vi "Day 7.vi"() -> ()   [LabVIEW 2021]
uses:
  <vilib>/Utility/file.llb/Read Delimited Spreadsheet (I64).vi
panel:
  out "Min Position":i32
  out "Input":i64[](array[numeric])
  out "Solution Min Fuel":i32
  in  "Input File":enum32{"example input", "input"}(radio)
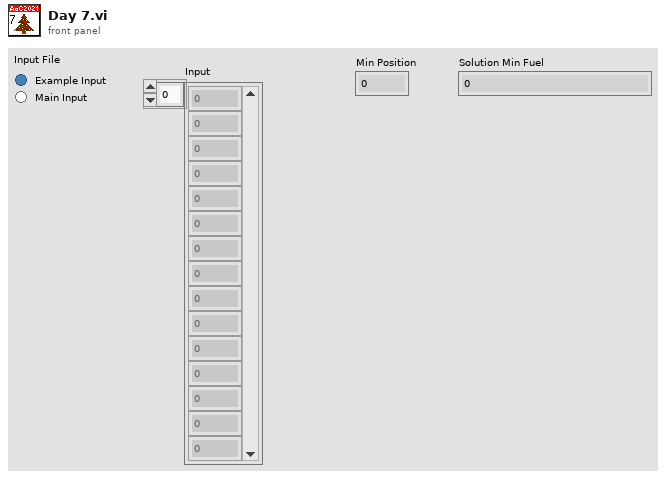
[diagram p1: front panel]
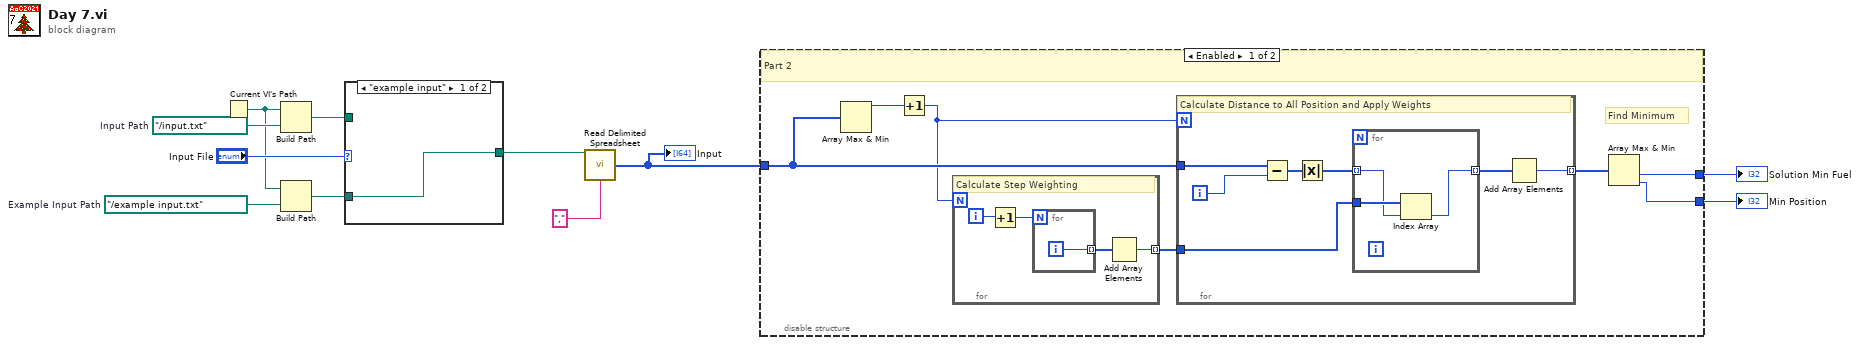
[diagram p0: block diagram]
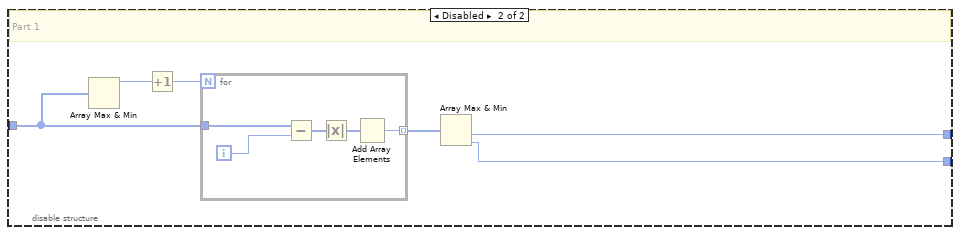
[diagram p3: hidden frame]
diagram:
  w10 = path "../example input.txt"  # Example Input Path
  w11 = path "../input.txt"  # Input Path
  n1 = Current VI's Path() -> (path=w5:path)
  n2 = Build Path(base path=w5, name or relative path=w11) -> (appended path=w8:path)
  n3 = Build Path(base path=w5, name or relative path=w10) -> (appended path=w7:path)
  n4 = case shown="\"example input\"" "Input File" {
    tunnel: w8 -> [_ w13]
    tunnel: w7 -> [w12 _]
    tunnel: [w12 w13] -> w6
    frame "example input" {
    }
    frame "input" {
    }
  }
  n5 = call-poly <vilib>:"Read Delimited Spreadsheet.vi"("file path (dialog if empty)"=w6, "delimiter (\\t)"="," ("delimiter (\\t)")) -> ("first row"=w1:i64[])  [unwired: 8 in, 5 out]
  "Input" <- w1
  n6 = disable-structure shown="Enabled" {
    disable-tunnel: w1 -> [w20 w41]
    disable-tunnel: [w17 w37] -> w3
    disable-tunnel: [w16 w36] -> w2
    frame Enabled {
      # "Find Minimum"
      # "Part 2"
      n7 = Array Max & Min(array=w20) -> (max value=w19:i64)  [unwired: 3 out]
      n8 = Increment(x=w19) -> (x+1=w15:i64)
      n9 = for {
        N: w15 -> [_]
        tunnel: [w21] -> w14 mode=indexing
        i -> [w24]
        # "Calculate Step Weighting"
        n10 = Increment(x=w24) -> (x+1=w23:i32)
        n11 = for {
          N: w23 -> [_]
          tunnel: [w25] -> w22 mode=indexing
          i -> [w25]
        }
        n12 = Add Array Elements(numeric array=w22) -> (sum=w21:i32)
      }
      n13 = for {
        N: w15 -> [_]
        tunnel: w20 -> [w32]
        tunnel: [w29] -> w18 mode=indexing
        tunnel: w14 -> [w27]
        i -> [w31]
        # "Calculate Distance to All Position and Apply Weights"
        n14 = Subtract(x=w32, y=w31) -> (x-y=w30:i64[])
        n15 = Absolute Value(x=w30) -> (abs(x)=w26:i64[])
        n16 = for {
          tunnel: w26 -> [w34] mode=indexing
          tunnel: [w33] -> w28 mode=indexing
          tunnel: w27 -> [w35]
          n17 = Index Array(array=w35, index=w34) -> (element=w33:i32)
        }
        n18 = Add Array Elements(numeric array=w28) -> (sum=w29:i32)
      }
      n19 = Array Max & Min(array=w18) -> (min value=w17:i32, min index (indices)=w16:i32)  [unwired: 2 out]
    }
    frame Disabled {
      # "Part 1"
      n20 = Array Max & Min(array=w41) -> (max value=w40:i64)  [unwired: 3 out]
      n21 = Increment(x=w40) -> (x+1=w39:i64)
      n22 = for {
        N: w39 -> [_]
        tunnel: w41 -> [w46]
        tunnel: [w43] -> w38 mode=indexing
        i -> [w45]
        n23 = Subtract(x=w46, y=w45) -> (x-y=w44:i64[])
        n24 = Absolute Value(x=w44) -> (abs(x)=w42:i64[])
        n25 = Add Array Elements(numeric array=w42) -> (sum=w43:i64)
      }
      n26 = Array Max & Min(array=w38) -> (min value=w37:i64, min index (indices)=w36:i32)  [unwired: 2 out]
    }
  }
  "Solution Min Fuel" <- w3
  "Min Position" <- w2
